vi "API BAROpen.vi"(10 "portNum":i32) -> (3 "DevOpen Return Value":bool)   [LabVIEW 2011, in "API READBC.lvlib"]
uses:
  API READBC.lvlib
  BarCodeAPI.dll
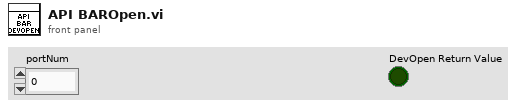
[diagram p1: front panel]
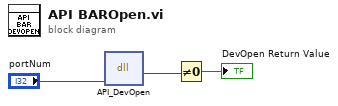
[diagram p0: block diagram]
diagram:
  n1 = dll-call lib="PTH1oabs CUsers\nAdministratorDesktop可重构机电平台项目DemoLabView基础APIBarCodeAPI.dll" fn="API_DevOpen"("portNum"="portNum") -> ("返回类型"=w2:i32)  [unwired: 4 in, 2 out]
  n2 = Not Equal To 0?(x=w2) -> (x != 0?=→"DevOpen Return Value":bool)
